vi "PROXY_destroy_queues.vi"(8 "error_in":errorcluster, 11 "all_config_info":T1) -> (0 "error_out":errorcluster)   [LabVIEW 2020]
uses:
  ini/typedef/PROXY_all_config_info.ctl
  ini/typedef/PROXY_main_ini_file.ctl
  typedef/PROXY_queue_refnums.ctl
  typedef/STATION_queue_element.ctl
  STATION/ST_SQL_sequence_state.ctl
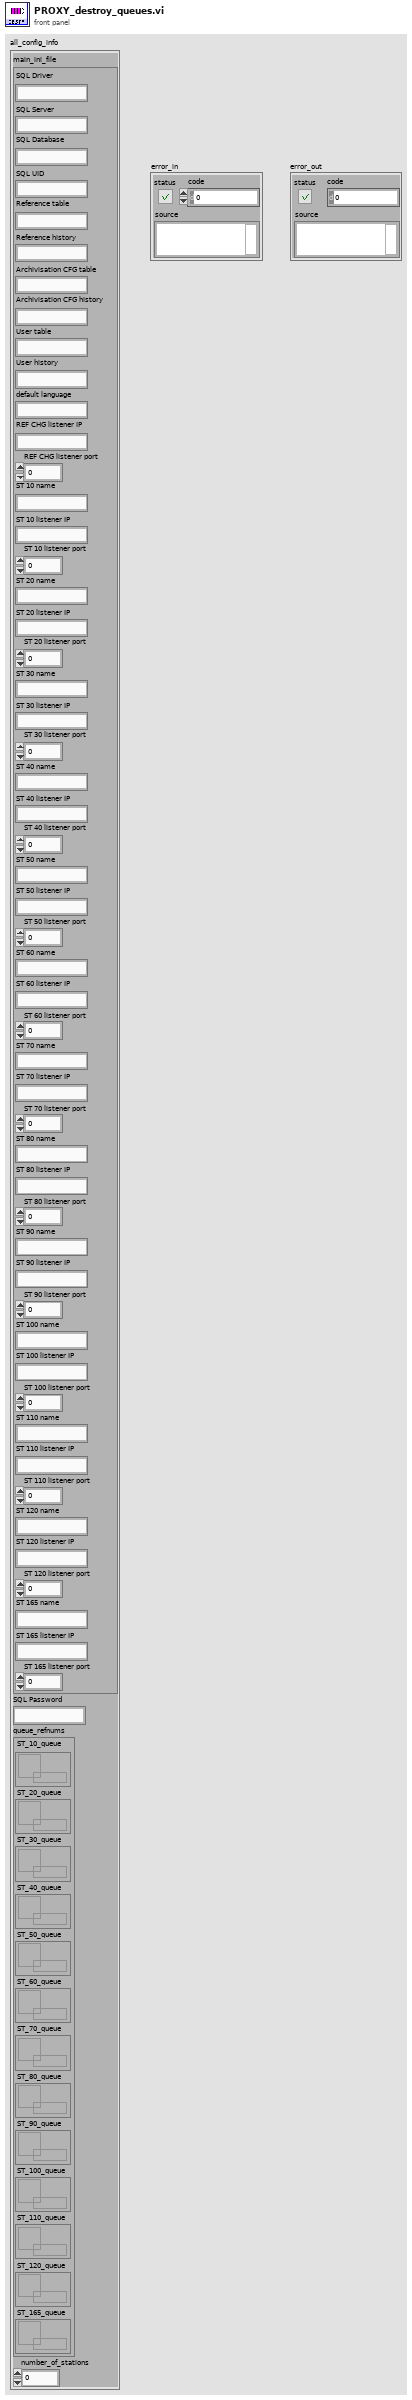
[diagram p1: front panel]
types:
  T1 = typedef "PROXY_all_config_info.ctl" = cluster{"main_ini_file":T2, "SQL Password":string, "queue_refnums":T3, "number_of_stations":i32}
  T2 = typedef "PROXY_main_ini_file.ctl" = cluster{"SQL Driver":string, "SQL Server":string, "SQL Database":string, "SQL UID":string, "Reference table":string, "Reference history":string, "Archivisation CFG table":string, "Archivisation CFG history":string, "User table":string, "User history":string, "default language":string, "REF CHG listener IP":string, "REF CHG listener port":u16, "ST 10 name":string, "ST 10 listener IP":string, "ST 10 listener port":u16, "ST 20 name":string, "ST 20 listener IP":string, "ST 20 listener port":u16, "ST 30 name":string, "ST 30 listener IP":string, "ST 30 listener port":u16, "ST 40 name":string, "ST 40 listener IP":string, "ST 40 listener port":u16, "ST 50 name":string, "ST 50 listener IP":string, "ST 50 listener port":u16, "ST 60 name":string, "ST 60 listener IP":string, "ST 60 listener port":u16, "ST 70 name":string, "ST 70 listener IP":string, "ST 70 listener port":u16, "ST 80 name":string, "ST 80 listener IP":string, "ST 80 listener port":u16, "ST 90 name":string, "ST 90 listener IP":string, "ST 90 listener port":u16, "ST 100 name":string, "ST 100 listener IP":string, "ST 100 listener port":u16, "ST 110 name":string, "ST 110 listener IP":string, "ST 110 listener port":u16, "ST 120 name":string, "ST 120 listener IP":string, "ST 120 listener port":u16, "ST 165 name":string, "ST 165 listener IP":string, "ST 165 listener port":u16}
  T3 = typedef "PROXY_queue_refnums.ctl" = cluster{"ST_10_queue":refnum<queue>, "ST_20_queue":refnum<queue>, "ST_30_queue":refnum<queue>, "ST_40_queue":refnum<queue>, "ST_50_queue":refnum<queue>, "ST_60_queue":refnum<queue>, "ST_70_queue":refnum<queue>, "ST_80_queue":refnum<queue>, "ST_90_queue":refnum<queue>, "ST_100_queue":refnum<queue>, "ST_110_queue":refnum<queue>, "ST_120_queue":refnum<queue>, "ST_165_queue":refnum<queue>}
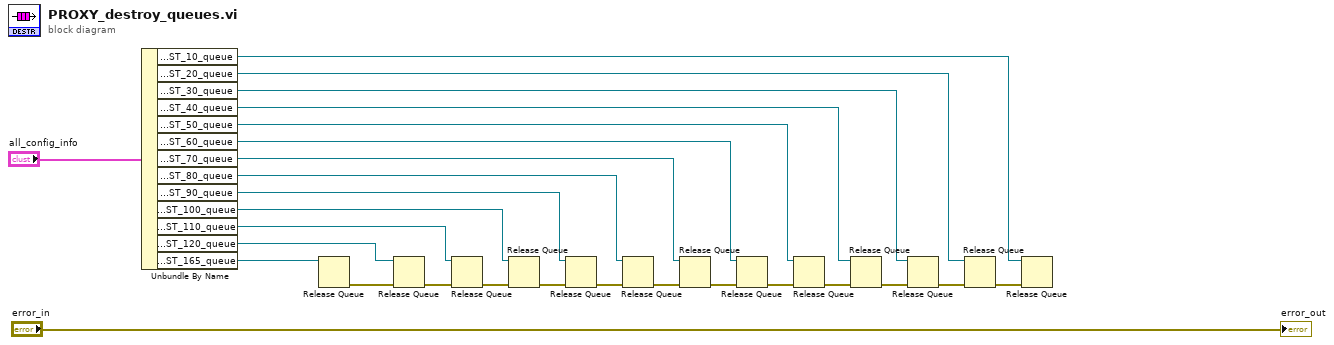
[diagram p0: block diagram]
diagram:
  n1 = Unbundle By Name("all_config_info") -> ("queue_refnums.ST_10_queue"=w27:refnum<queue>, "queue_refnums.ST_20_queue"=w25:refnum<queue>, "queue_refnums.ST_30_queue"=w24:refnum<queue>, "queue_refnums.ST_40_queue"=w12:refnum<queue>, "queue_refnums.ST_50_queue"=w11:refnum<queue>, "queue_refnums.ST_60_queue"=w10:refnum<queue>, "queue_refnums.ST_70_queue"=w9:refnum<queue>, "queue_refnums.ST_80_queue"=w8:refnum<queue>, "queue_refnums.ST_90_queue"=w7:refnum<queue>, "queue_refnums.ST_100_queue"=w6:refnum<queue>, "queue_refnums.ST_110_queue"=w5:refnum<queue>, "queue_refnums.ST_120_queue"=w4:refnum<queue>, "queue_refnums.ST_165_queue"=w2:refnum<queue>)
  n2 = Release Queue(queue=w2) -> (error out=w1:errorcluster)  [unwired: 2 in, 2 out]
  n3 = Release Queue(queue=w4, error in (no error)=w1) -> (error out=w3:errorcluster)  [unwired: 1 in, 2 out]
  n4 = Release Queue(queue=w5, error in (no error)=w3) -> (error out=w13:errorcluster)  [unwired: 1 in, 2 out]
  n5 = Release Queue(queue=w6, error in (no error)=w13) -> (error out=w14:errorcluster)  [unwired: 1 in, 2 out]
  n6 = Release Queue(queue=w7, error in (no error)=w14) -> (error out=w15:errorcluster)  [unwired: 1 in, 2 out]
  n7 = Release Queue(queue=w8, error in (no error)=w15) -> (error out=w19:errorcluster)  [unwired: 1 in, 2 out]
  n8 = Release Queue(queue=w9, error in (no error)=w19) -> (error out=w16:errorcluster)  [unwired: 1 in, 2 out]
  n9 = Release Queue(queue=w10, error in (no error)=w16) -> (error out=w17:errorcluster)  [unwired: 1 in, 2 out]
  n10 = Release Queue(queue=w11, error in (no error)=w17) -> (error out=w20:errorcluster)  [unwired: 1 in, 2 out]
  n11 = Release Queue(queue=w12, error in (no error)=w20) -> (error out=w18:errorcluster)  [unwired: 1 in, 2 out]
  n12 = Release Queue(queue=w24, error in (no error)=w18) -> (error out=w21:errorcluster)  [unwired: 1 in, 2 out]
  n13 = Release Queue(queue=w25, error in (no error)=w21) -> (error out=w22:errorcluster)  [unwired: 1 in, 2 out]
  n14 = Release Queue(queue=w27, error in (no error)=w22) -> ()  [unwired: 1 in, 3 out]
  "error_out" <- "error_in"
